vi "Read Interface_type.vi"(8 "error in (no error)":errorcluster, 11 "_Driver_interaction in":refnum<class "_Driver_interaction.lvclass">) -> (0 "error out":errorcluster, 2 "Interface_type":T1="DALI", 3 "_Driver_interaction out":refnum<class "_Driver_interaction.lvclass">)   [LabVIEW 2014, in "Driver_interaction.lvlib" / "_Driver_interaction.lvclass"]
uses:
  _Driver_interaction.lvclass
  Controls/Interface_type.ctl
  _Driver_interaction.lvclass/_Driver_interaction.ctl
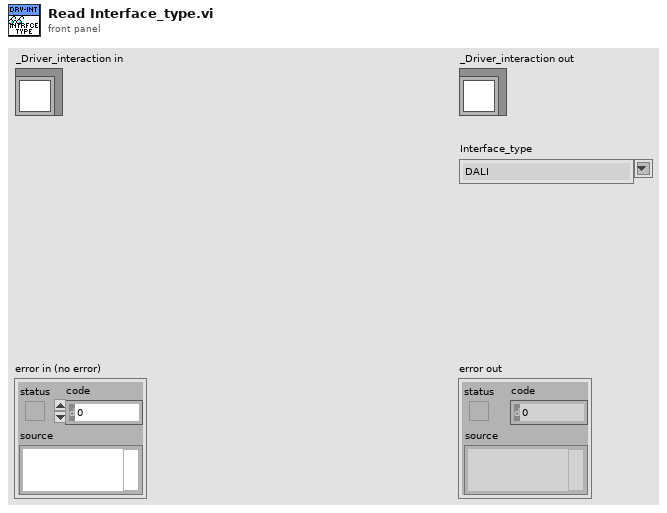
[diagram p1: front panel]
types:
  T1 = typedef "Driver_interaction.lvlib/_Driver_interaction.lvclass/Interface_type.ctl" = string
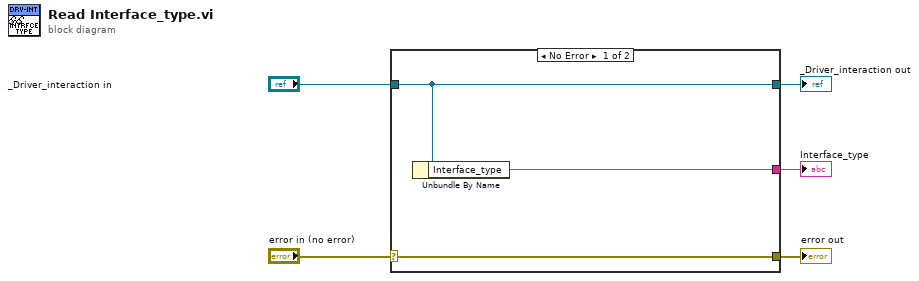
[diagram p0: block diagram]
diagram:
  n1 = case shown="No Error" "error in (no error)" {
    selector: "error in (no error)" -> [w8 w9]
    tunnel: [w8 w9] -> w4
    tunnel: [w7 w10] -> w2
    tunnel: "_Driver_interaction in" -> [w7 w10]
    tunnel: [w6 _] -> w1
    frame No Error {
      n2 = Unbundle By Name(w7) -> ("Interface_type"=w6:T1)
    }
    frame Error {
    }
  }
  "error out" <- w4
  "_Driver_interaction out" <- w2
  "Interface_type" <- w1
